vi "Show_Temperature.vi"() -> ()   [LabVIEW 2010]
panel:
  out "Temperature":cluster{timestamp[], dbl[]}(graph)
  out "error out":errorcluster
  in  "error in":errorcluster
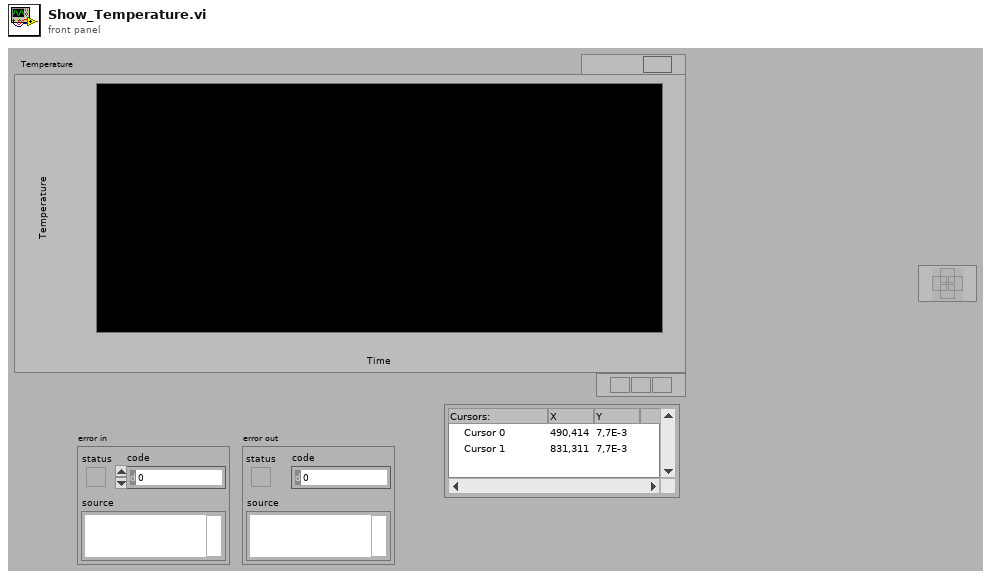
[diagram p1: front panel]
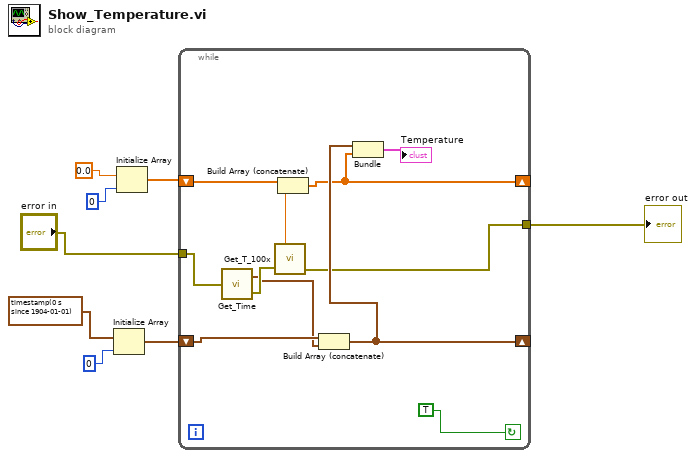
[diagram p0: block diagram]
diagram:
  n1 = Initialize Array(timestamp(0 s since 1904-01-01), 0) -> (w2:timestamp[])
  n2 = Initialize Array(0.0, 0) -> (w6:dbl[])
  n3 = while {
    shift-right: [w14] -> _
    shift-left: w6 -> [w19]
    shift-right: [w15] -> _
    shift-left: w2 -> [w17]
    tunnel: "error in" -> [w11]
    tunnel: [w12] -> w7
    stop <- TRUE continue-if-true
    n4 = call "Get_Time.vi"("error in"=w11) -> ("error in 2"=w10:errorcluster, "seconds since 1Jan1904"=w9:timestamp)
    n5 = call "Get_T_100x.vi"("error in"=w10) -> ("error out"=w12:errorcluster, "Temperature Mean"=w18:dbl)  [unwired: 1 in, 1 out]
    n6 = Build Array (concatenate)(w19, w18) -> (w14:dbl[])
    n7 = Build Array (concatenate)(w17, w9) -> (w15:timestamp[])
    n8 = Bundle(w15, w14) -> (→"Temperature":cluster{timestamp[], dbl[]})  [unwired: 1 in]
  }
  "error out" <- w7
